vi "equals.vi"(8 "error in (no error)":errorcluster, 10 "object 2":refnum<class>, 11 "pRectangle in":refnum<class "pRectangle.lvclass">) -> (0 "error out":errorcluster, 2 "equal?":bool, 3 "pRectangle out":refnum<class "pRectangle.lvclass">)   [LabVIEW 2018, in "pRectangle.lvclass"]
uses:
  pRectangle.lvclass
  pRectangle.lvclass/pRectangle.ctl
  Shape Class/pShape.lvclass
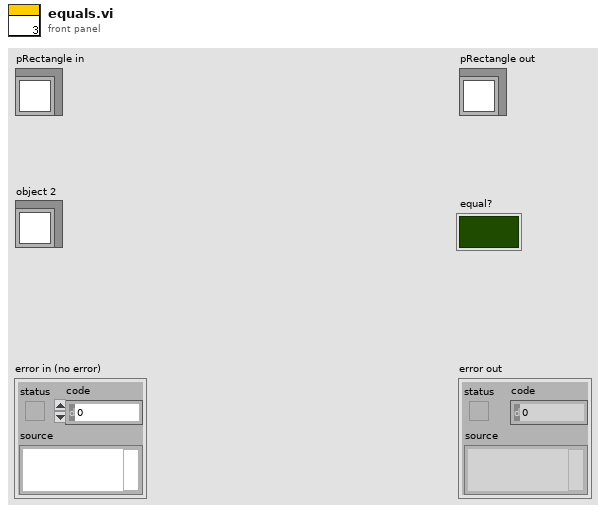
[diagram p1: front panel]
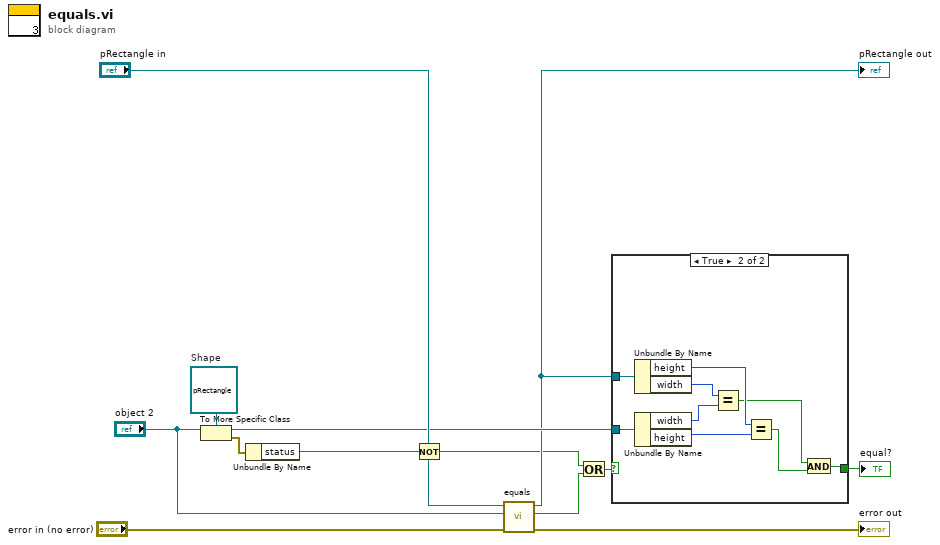
[diagram p0: block diagram]
diagram:
  w9 = refnum<class "pRectangle.lvclass"> refnum  # Shape
  n1 = To More Specific Class(target class=w9, reference="object 2") -> (specific class reference=w3:refnum<class "pRectangle.lvclass">, error out=w10:errorcluster)  [unwired: 1 in]
  n2 = Unbundle By Name(w10) -> ("status"=w6:bool)
  n3 = Not(x=w6) -> (.not. x?=w1:bool)
  n4 = call-parent "equals.vi"("error in (no error)"="error in (no error)", "object 2"="object 2", "pShape in"="pRectangle in") -> ("error out"=→"error out":errorcluster, "equal?"=w7:bool, "pShape out"=w2:refnum<class "pRectangle.lvclass">)  [unwired: 6 in]
  "pRectangle out" <- w2
  n5 = Or(x=w1, y=w7) -> (x .or. y?=w5:bool)
  n6 = case shown="True" w5 {
    selector: w5 -> [w14 _]
    tunnel: [w14 w17] -> w4
    tunnel: w3 -> [_ w22]
    tunnel: w2 -> [_ w23]
    frame False {
    }
    frame True {
      n7 = Unbundle By Name(w23) -> ("height"=w19:i32, "width"=w21:i32)
      n8 = Unbundle By Name(w22) -> ("width"=w20:i32, "height"=w18:i32)
      n9 = Equal?(x=w21, y=w20) -> (x = y?=w16:bool)
      n10 = Equal?(x=w19, y=w18) -> (x = y?=w15:bool)
      n11 = And(x=w16, y=w15) -> (x .and. y?=w17:bool)
    }
  }
  "equal?" <- w4
